vi "kvCanObjBufWrite.vi"(0 "Channel Handle (input only)":i32, 1 "Object Handle":i32, 2 "Message Id":i32, 3 "Message Data":u8[](array[numeric]), 4 "DLC":u8, 5 "Remote Request":bool, 6 "Standard 11-bit Id":bool, 7 "error in (no error)":errorcluster, 8 "Single Shot":bool, 9 "Extended 29-bit Id":bool, 10 "Error Frame":bool, 11 "FD Frame":bool, 12 "Wakeup":bool, 13 "Bit Rate Switch":bool) -> (22 "Channel Handle (output only)":i32, 25 "error out":errorcluster)   [LabVIEW 2022 SP3]
doc: "Defines the message content to be transmitted by the object buffer."
uses:
  canlib32.dll
panel:
  # "8"
  # "16"
  # "24"
  # "32"
  # "40"
  # "48"
  # "56"
  # "64"
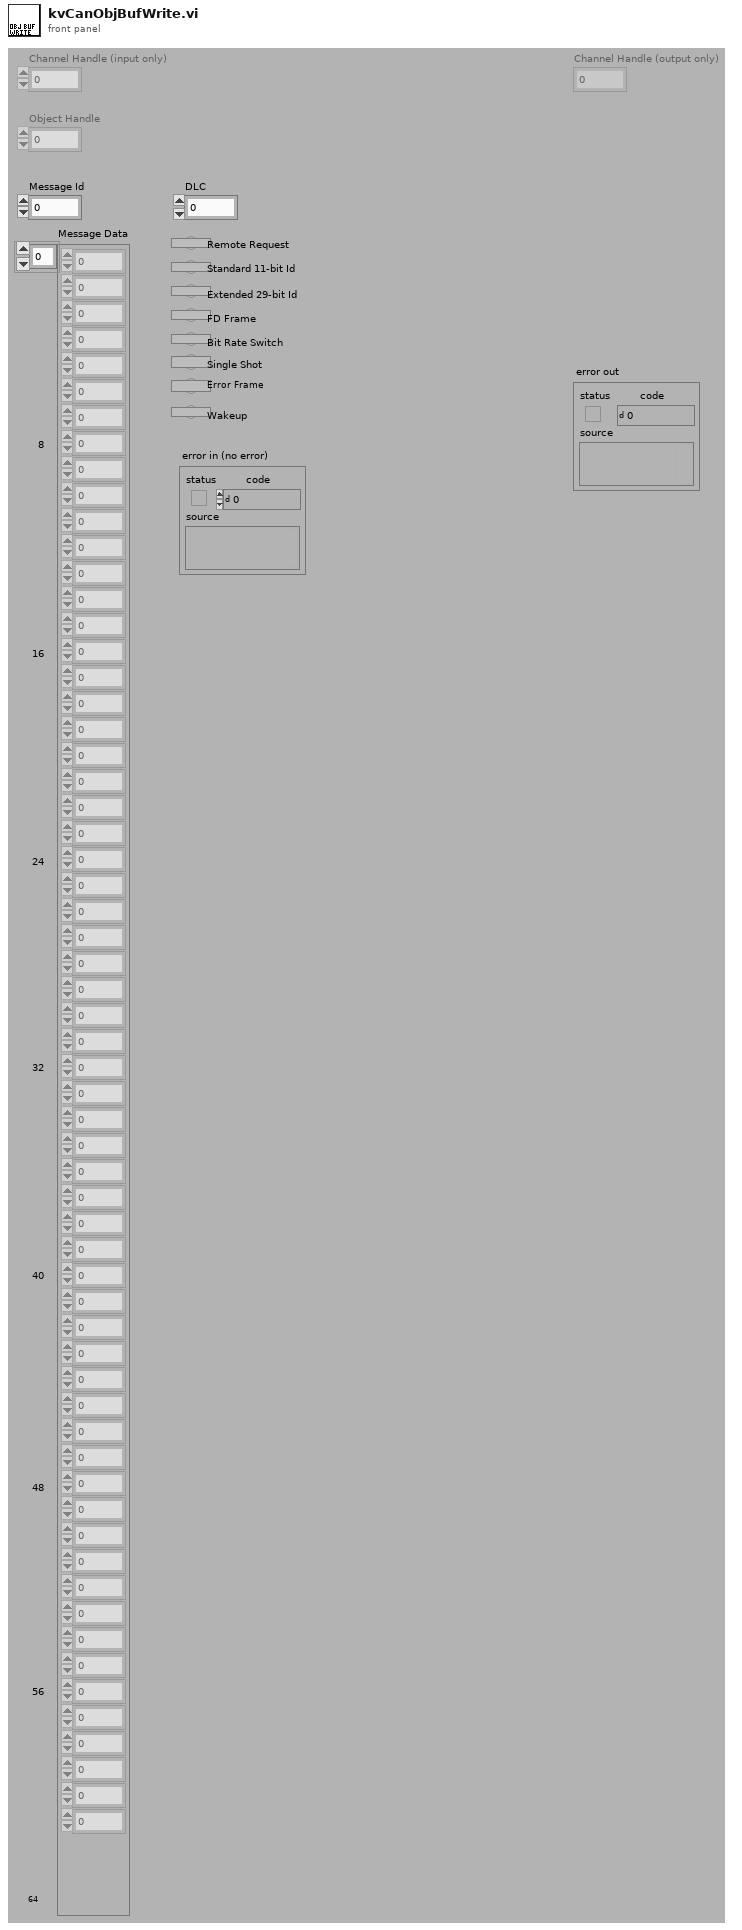
[diagram p1: front panel]
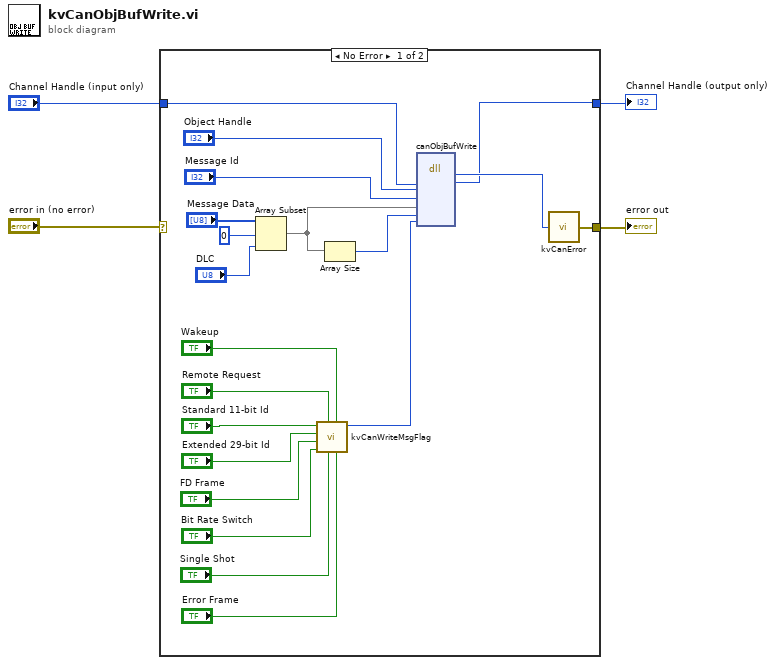
[diagram p0: block diagram]
diagram:
  n1 = case shown="No Error" "error in (no error)" {
    selector: "error in (no error)" -> [_ w25]
    tunnel: "Channel Handle (input only)" -> [w21 w26]
    tunnel: [w22 w26] -> w2
    tunnel: [w24 w25] -> w1
    frame No Error {
      n2 = Array Subset(array="Message Data", index=0, length="DLC") -> (w16:u8[])
      n3 = call "kvCanWriteMsgFlag.vi"("Error Frame"="Error Frame", "Wakeup"="Wakeup", "Single Shot"="Single Shot", "Remote Request"="Remote Request", "Bit Rate Switch"="Bit Rate Switch", "FD Frame"="FD Frame", "Extended 29-bit Id"="Extended 29-bit Id", "Standard 11-bit Id"="Standard 11-bit Id") -> ("Flag Value"=w18:u32)  [unwired: 3 in]
      n4 = Array Size(array=w16) -> (size(s)=w15:i32)
      n5 = dll-call lib="canlib32.dll" fn="canObjBufWrite"("chan"=w21, "idx"="Object Handle", "id"="Message Id", "msg"=w16, "dlc"=w15, "flags"=w18) -> (w23:i32, "chan"=w22:i32)  [unwired: 8 in, 2 out]
      n6 = call "kvCanError.vi"("error code"=w23) -> ("error out"=w24:errorcluster)
    }
    frame Error {
    }
  }
  "Channel Handle (output only)" <- w2
  "error out" <- w1
